vi "GV_AutoscaleCalcRange.vi"(8 "BottomVal":dbl, 9 "TopVal":dbl, 10 "Min_data":dbl, 11 "Max_data":dbl) -> (1 "Min Setting":dbl, 3 "Max Setting":dbl)   [LabVIEW 2020, in "Sgraph_lib_V1.lvlib" / "Gviewer.lvclass"]
doc: "Andre Koelewijn, 17 aug 2021\n\nThis VI will calculate the Gain and Offset value of a trace based upon the \nMax graph range of +1 and Min graph range of -1"
uses:
  Gviewer.lvclass
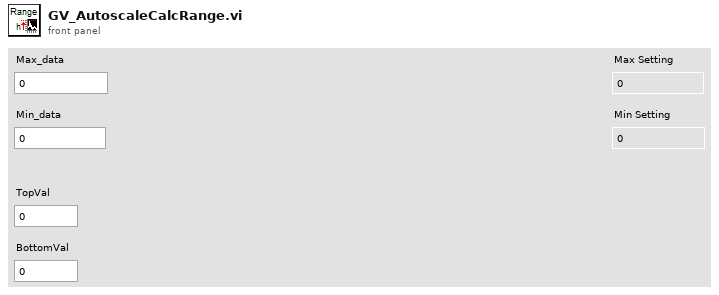
[diagram p1: front panel]
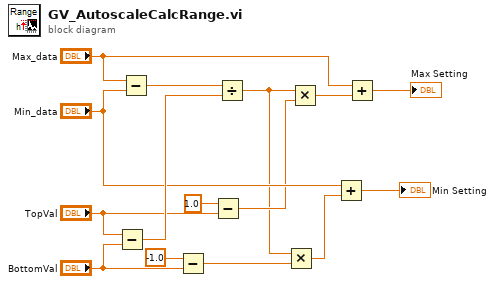
[diagram p0: block diagram]
diagram:
  n1 = Subtract(x="TopVal", y="BottomVal") -> (x-y=w14:dbl)
  n2 = Subtract(x="Max_data", y="Min_data") -> (x-y=w15:dbl)
  n3 = Subtract(x=-1.0, y="BottomVal") -> (x-y=w11:dbl)
  n4 = Subtract(x=1.0, y="TopVal") -> (x-y=w5:dbl)
  n5 = Divide(x=w15, y=w14) -> (x/y=w4:dbl)
  n6 = Multiply(x=w4, y=w11) -> (x*y=w9:dbl)
  n7 = Multiply(x=w4, y=w5) -> (x*y=w3:dbl)
  n8 = Add(x="Min_data", y=w9) -> (x+y=→"Min Setting":dbl)
  n9 = Add(x="Max_data", y=w3) -> (x+y=→"Max Setting":dbl)
